vi "Sine Wave.vi"(5 "숫자형":i32) -> (1 "사인파":dbl)   [LabVIEW 2011]
uses:
  <vilib>/ptbypt/NI_PtbyPt.lvlib
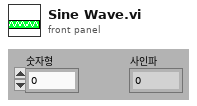
[diagram p1: front panel]
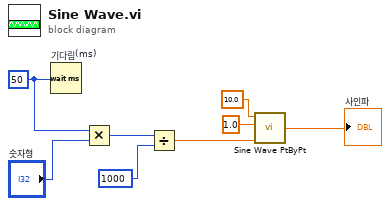
[diagram p0: block diagram]
diagram:
  w5 = u32 50 ("milliseconds to wait")
  n1 = Wait (ms) "기다림(ms)"(milliseconds to wait=w5) -> ()  [unwired: 1 out]
  n2 = Multiply(x=w5, y="숫자형") -> (x*y=w7:u32)
  n3 = Divide(x=w7, y=u32 1000) -> (x/y=w8:dbl)
  n4 = call <vilib>:"Sine Wave PtByPt.vi"("time"=w8, "frequency"=1.0 ("f"), "amplitude"=10.0) -> ("sine wave"=→"사인파":dbl)  [unwired: 1 in]
